vi "stopAllMotion.vi"(8 "error in (no error)":errorcluster, 11 "DomeController in":refnum<class "DomeController.lvclass">) -> (0 "error out":errorcluster, 3 "DomeController out":refnum<class "DomeController.lvclass">)   [LabVIEW 2016, in "DomeController.lvclass"]
uses:
  DomeController.lvclass
  domeCommunicator/ComTypedefs/commands.ctl
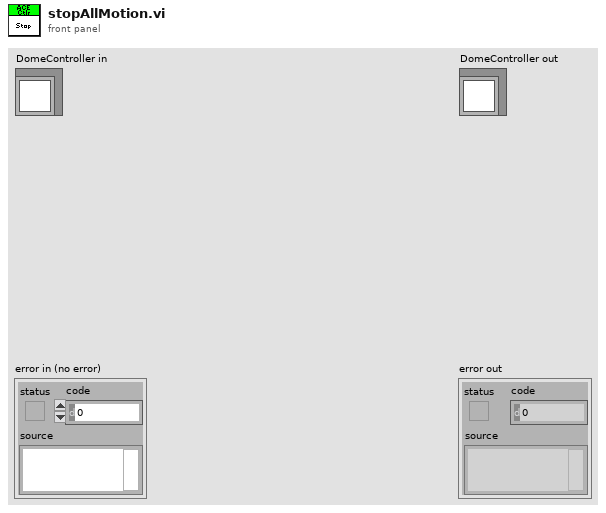
[diagram p1: front panel]
types:
  T1 = typedef "commands.ctl" = enum16{"StopAllMotion", "CloseMainDoor", "OpenMainDoor", "CloseDropoutDoor", "OpenDropoutDoor", "SynchronizedOpen", "SynchronizedClose", "AutoShutDownOn", "AutoShutDownOff", "RainOn", "RainOff", "CloudSensorOn", "CloudSensorOff", "RotateToHomePosition", "MoveToAzimuth", "SetTolerance", "DefineHomePosition", "HighSpeedThreshold", "SetCoast", "SetEncoderCountFor360", "SetWatchDogTimer", "SetReverseDirectionMotionDelay", "SaveCurrentConfiguration"}
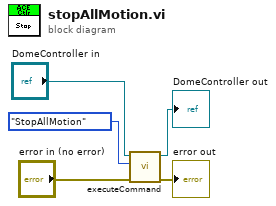
[diagram p0: block diagram]
diagram:
  n1 = call "executeCommand.vi"("error in (no error)"="error in (no error)", "commands"=commands."StopAllMotion", "DomeController in"="DomeController in") -> ("error out"=→"error out":errorcluster, "DomeController out"=→"DomeController out":refnum<class "DomeController.lvclass">)  [unwired: 7 in]
